vi "SetPrecision.vi"(8 "error in":errorcluster, 10 "Precision":u8=6, 11 "Decimal in":refnum<class "Decimal.lvclass">) -> (0 "error out":errorcluster, 3 "Decimal out":refnum<class "Decimal.lvclass">)   [LabVIEW 2021, in "ProligentXMLGenerator.lvlib" / "Decimal.lvclass"]
uses:
  Decimal.lvclass
  Decimal.lvclass/Decimal.ctl
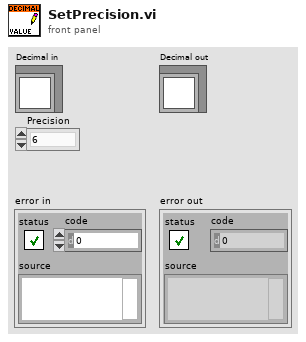
[diagram p1: front panel]
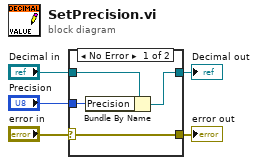
[diagram p0: block diagram]
diagram:
  n1 = case shown="No Error" "error in" {
    selector: "error in" -> [w6 w10]
    tunnel: "Decimal in" -> [w9 w11]
    tunnel: [w8 w11] -> w4
    tunnel: "Precision" -> [w7 _]
    tunnel: [w6 w10] -> w2
    frame No Error {
      n2 = Bundle By Name(cluster=w9, "Precision"=w7) -> (w8:refnum<class "Decimal.lvclass">)
    }
    frame Error {
    }
  }
  "error out" <- w2
  "Decimal out" <- w4
